vi "testIR.vi"() -> ()   [LabVIEW 2020]
uses:
  <vilib>/DAQmx/write.llb/DAQmx Write (Analog 2D DBL NChan NSamp).vi
  <vilib>/Utility/file.llb/Read Delimited Spreadsheet (DBL).vi
  <vilib>/DAQmx/miscellaneous.llb/DAQmx Fill In Error Info.vi
panel:
  out "Measured temperatures":dbl[](array[numeric])
  out "Input XY":i32[](array[numeric])
  in  "Desired temperature":dbl=30.0
  out "Input array":dbl[](array[numeric])
  in  "IR intensity value":dbl=10000.0
  in  "STIMULATE":bool
  out "Null Y output":dbl
  out "Null X output":dbl
  in  "LASER Intensity (%)":dbl=100.0 format="%#_13g"
  in  "Y input":i32=100
  in  "X input":i32=100
  out "Max. LASER Power (W)":dbl
  in  "Cycle Time (ms)":i32=50
  out "irData":dbl[](array[numeric])
  out "Temperature Measurements\n(Intensity Graph)":T1(graph)
  out "Intensity Graph":dbl[][](graph)
  out "Temperature array":dbl[][](array[numeric])
  in  "Temperature Range (High)":dbl=45.0
  in  "Temperature Range (Low)":dbl=20.0
  out "heatY":i32
  out "heatX":i32
  out "Deliver stimulation?":i32
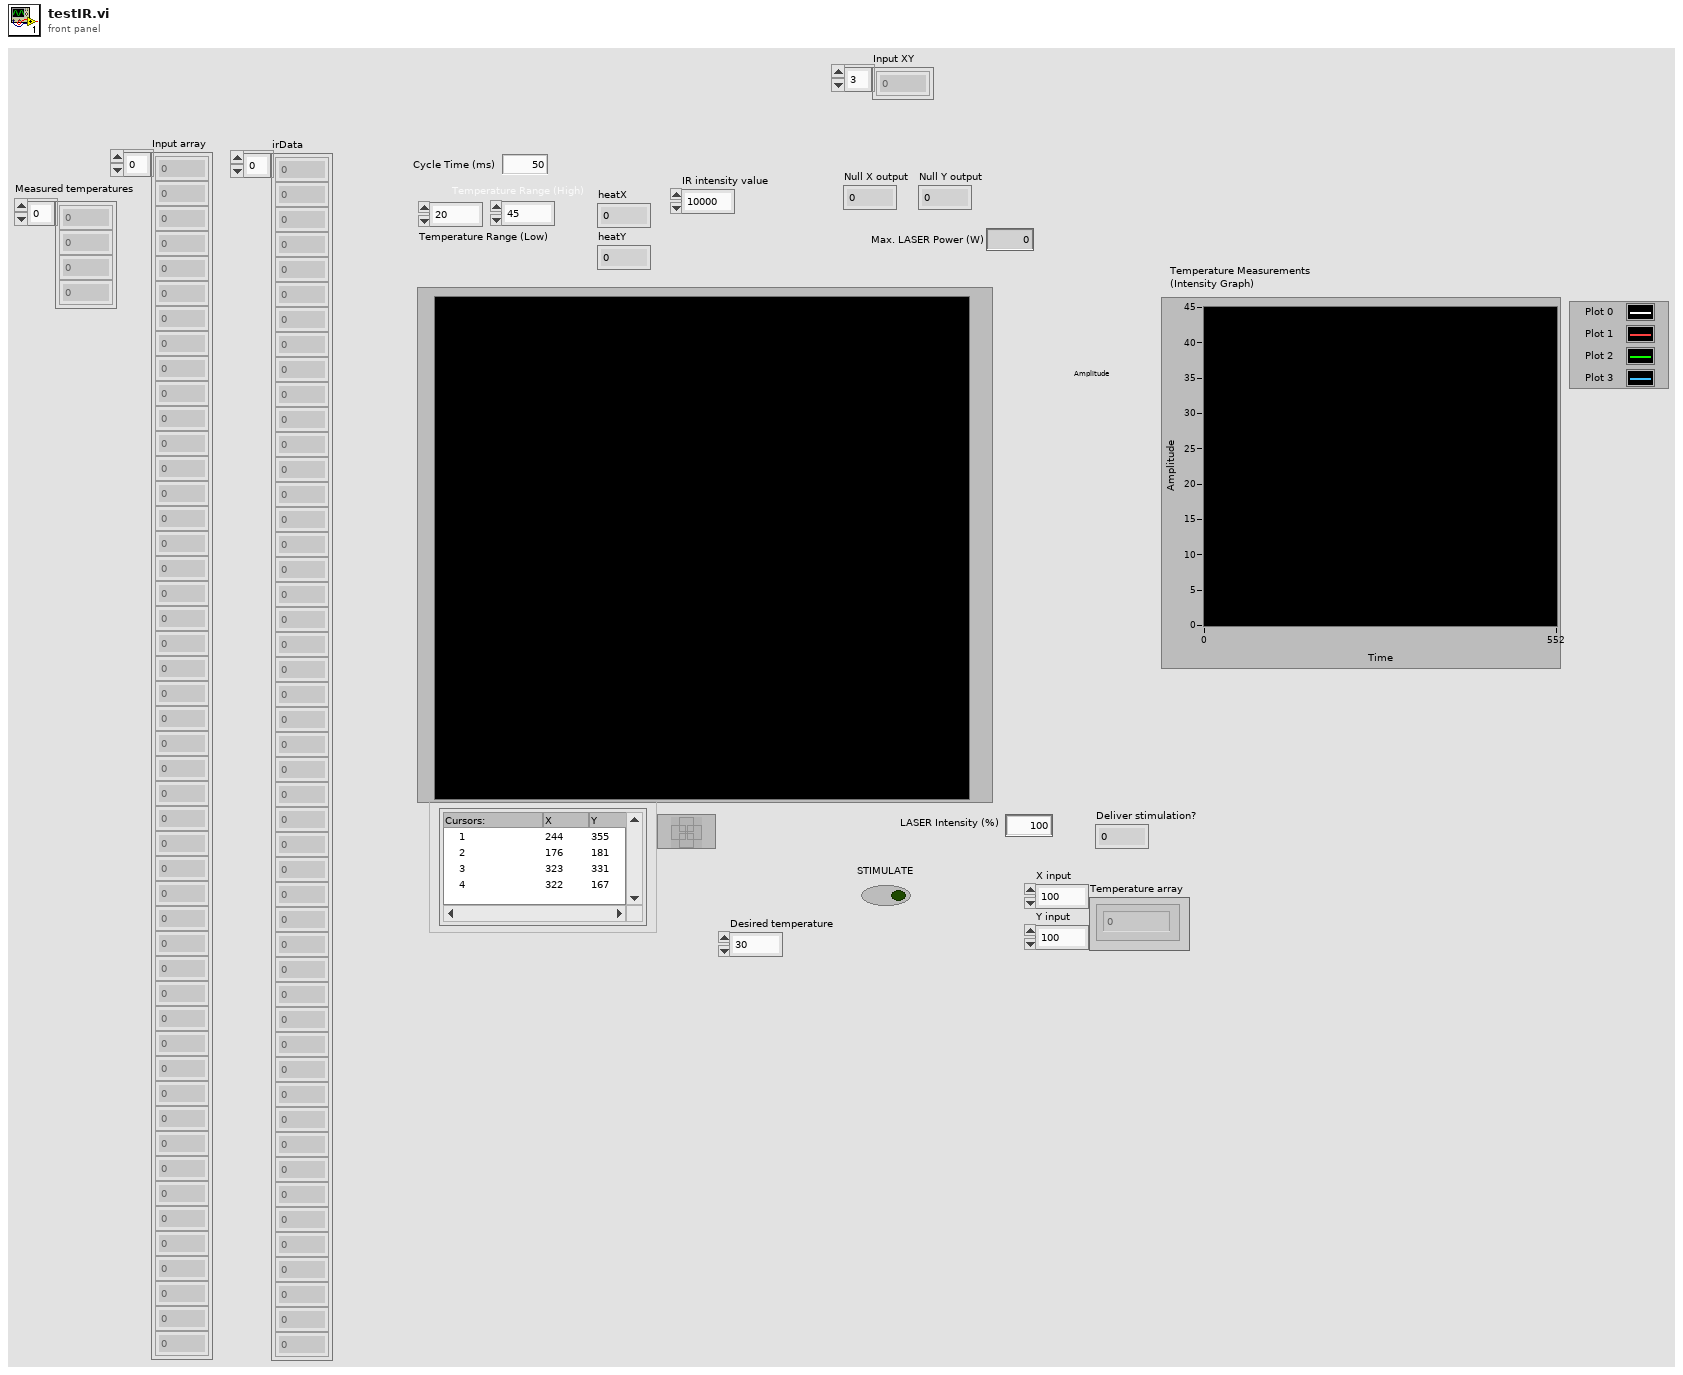
[diagram p1: front panel]
types:
  T1 = cluster{"[0]":dbl, "[1]":dbl, "[2]":dbl, "[3]":dbl, "[4]":dbl, "[5]":dbl, "[6]":dbl, "[7]":dbl, "[8]":dbl}
  T2 = enum16{"fire", "rainbow", "gray", "inverse gray", "ice", "original"}
  T3 = enum16{"open", "replace", "create", "open or create", "replace or create", "replace or create with confirmation"}
  T4 = enum16{"big-endian, network order", "native, host order", "little-endian"}
  T5 = typedef "IR GALVO Cal Data.ctl" = cluster{"G1X":dbl[][], "G1Y":dbl[][], "G2X":dbl[][], "G2Y":dbl[][], "G3X":dbl[][], "G3Y":dbl[][], "G4X":dbl[][], "G4Y":dbl[][], "G1 Intensity":dbl[][], "G2 Intensity":dbl[][], "G3 Intensity":dbl[][], "G4 Intensity":dbl[][], "L1 POWER":dbl[]}
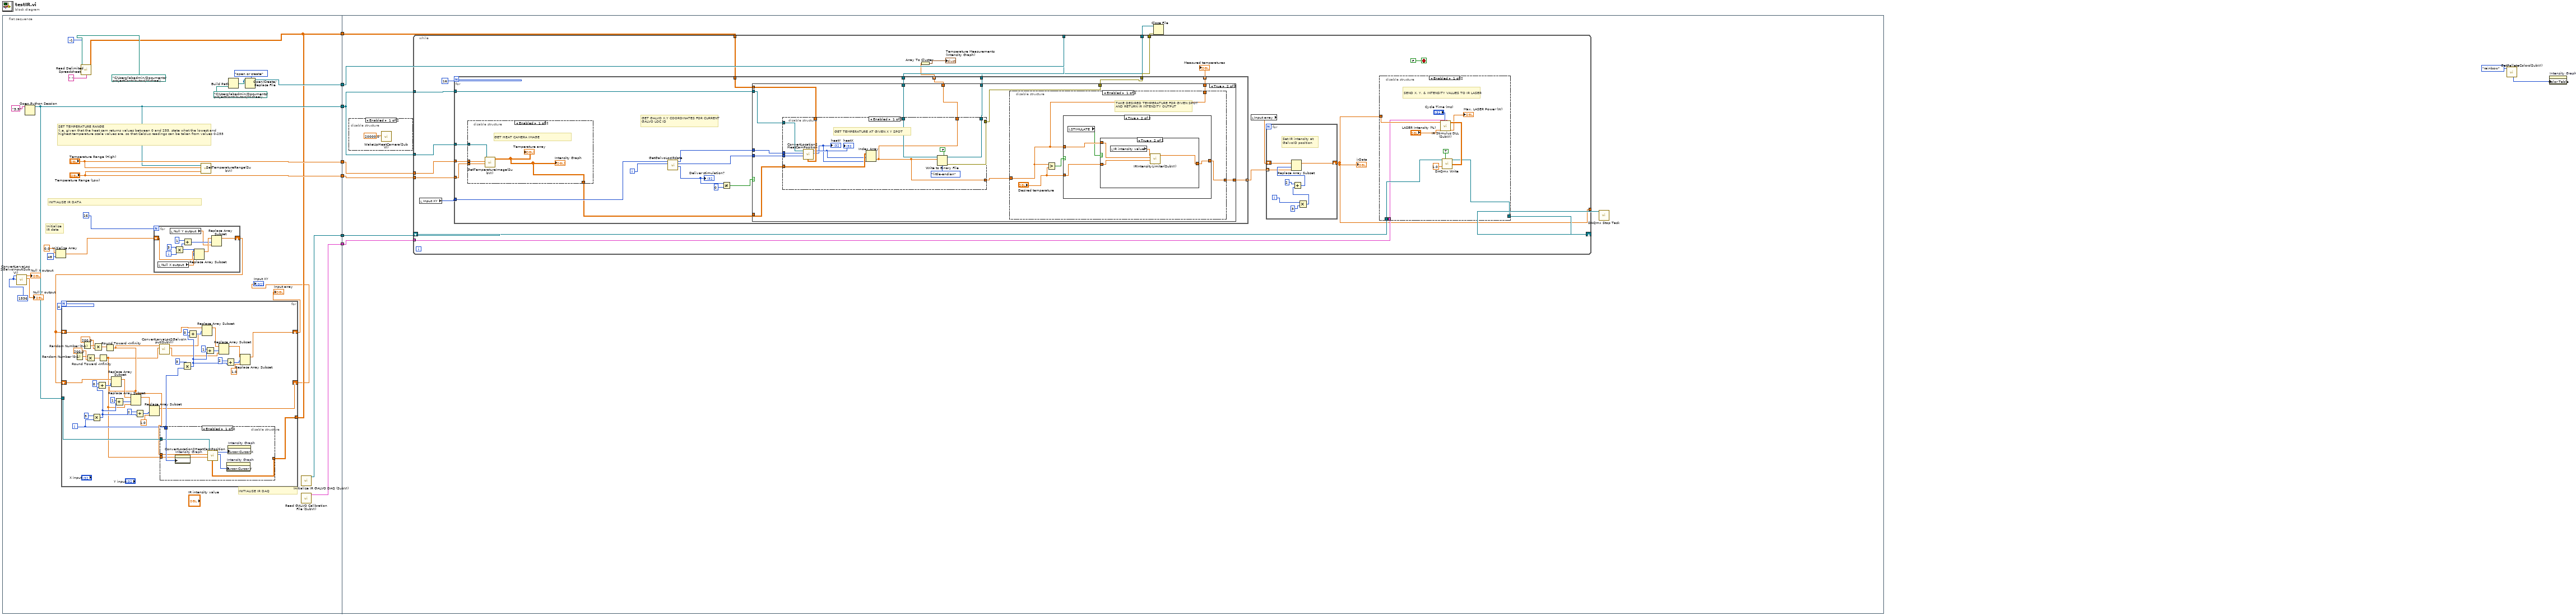
[diagram p0: block diagram]
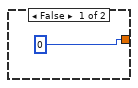
[diagram p4: hidden frame]
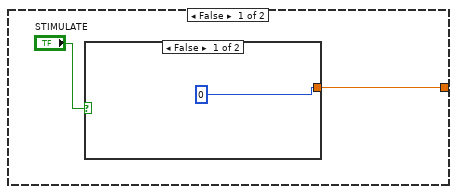
[diagram p6: hidden frame]
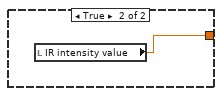
[diagram p7: hidden frame]
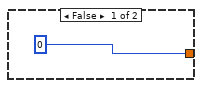
[diagram p8: hidden frame]
diagram:
  n1 = flat-sequence {
    tunnel: [w13] -> w7
    tunnel: ["Temperature Range (High)"] -> w6
    tunnel: ["Temperature Range (Low)"] -> w5
    tunnel: [w25] -> w4
    tunnel: [w23] -> w3
    tunnel: [w12] -> w2
    tunnel: [w16] -> w1
    tunnel: w7 -> [w93]
    tunnel: w6 -> [w92]
    tunnel: w5 -> [w91]
    tunnel: w4 -> [w99]
    tunnel: w3 -> [w98]
    tunnel: w2 -> [w97]
    tunnel: w1 -> [w96]
    frame #0 {
      w24 = 1536 ("X input")
      # "INITIALISE IR DAQ"
      # "INITIALISE IR DATA"
      # "SET TEMPERATURE RANGE\n(i.e. given that the heat cam returns values between 0 and 255, state what the lowest and highest temperature scale values are, so that Celsius readings can be taken from values 0-255"
      # "Initialise\nIR data"
      n2 = call "ConvertLarvaLoc2GalvoInput(SubVI).vi"("Y input"=w24, "X input"=w24) -> ("Y output"=→"Null Y output":dbl, "X output"=→"Null X output":dbl)  [unwired: 7 in, 1 out]
      n3 = Open Python Session(python version="3.9" ("Python version")) -> (session out=w13:refnum<k35>)  [unwired: 2 in, 1 out]
      n4 = Initialize Array(0.0 ("element"), 48 ("dimension size")) -> (w33:dbl[])
      n5 = call-poly <vilib>:"Read Delimited Spreadsheet.vi"("file path (dialog if empty)"=path "C:/Users/labadmin/Documents/projectContributors/Michael/multi-larva-cl-behavior-detection/LabViewSourceCode/heatCameraPythonCode/transformationMatrix.csv", "number of rows (all:-1)"=-1, "delimiter (\\t)"=" " ("delimiter (\\t)")) -> ("all rows"=w12:dbl[][])  [unwired: 7 in, 5 out]
      n6 = for {
        N: 16 -> [_]
        shift-right: [w37] -> w11
        shift-left: w33 -> [w41]
        i -> [w43]
        n7 = local read "Null X output"() -> (w36:dbl)
        n8 = local read "Null Y output"() -> (w35:dbl)
        n9 = Multiply(x=3, y=w43) -> (x*y=w40:i32)
        n10 = Add(x=1, y=w40) -> (x+y=w38:i32)
        n11 = Replace Array Subset(array=w41, new element=w36, index=w40) -> (w39:dbl[])
        n12 = Replace Array Subset(array=w39, new element=w35, index=w38) -> (w37:dbl[])
      }
      n13 = for {
        N: 4 -> [_]
        shift-right: [w82] -> w15
        shift-left: w11 -> [w79]
        tunnel: w13 -> [w66]
        tunnel: w12 -> [w61]
        shift-right: [w46] -> w10
        shift-left: w11 -> [w50]
        i -> [w48]
        n14 = Random Number (0-1)() -> (number: 0 to 1=w67:dbl)
        n15 = Random Number (0-1)() -> (number: 0 to 1=w70:dbl)
        n16 = Multiply(x=w67, y=200.0) -> (x*y=w65:dbl)
        n17 = Multiply(x=3, y=w48) -> (x*y=w59:i32)
        n18 = Multiply(x=w70, y=200.0) -> (x*y=w64:dbl)
        n19 = Add(x=0, y=w59) -> (x+y=w54:i32)
        n20 = Round Toward -Infinity(1:w65) -> (0:w45:dbl)
        n21 = Round Toward -Infinity(1:w64) -> (0:w49:dbl)
        n22 = Replace Array Subset(array=w50, new element=w49, index=w54) -> (w51:dbl[])
        n23 = Add(x=1, y=w59) -> (x+y=w56:i32)
        n24 = Replace Array Subset(array=w51, new element=w45, index=w56) -> (w52:dbl[])
        n25 = Add(x=2, y=w59) -> (x+y=w58:i32)
        n26 = Replace Array Subset(array=w52, new element=1.0 ("new element/subarray"), index=w58) -> (w46:dbl[])
        n27 = call "ConvertLarvaLoc2GalvoInput(SubVI).vi"("Y input"=w45, "X input"=w49) -> ("Y output"=w62:dbl, "X output"=w63:dbl)  [unwired: 7 in, 1 out]
        n28 = disable-structure shown="Enabled" {
          disable-tunnel: w48 -> [w90 _]
          disable-tunnel: w66 -> [w89 _]
          disable-tunnel: w61 -> [w86 _]
          disable-tunnel: w49 -> [w85 _]
          disable-tunnel: w45 -> [w84 _]
          frame Enabled {
            n29 = property on="Intensity Graph" class="IntGraph (strict)"("Active Cursor"=w90) -> ()  [unwired: 2 in, 2 out]
            n30 = call "ConvertLocation2HeatCamPosition.vi"("Transformation matrix"=w86, "yLoc"=w84, "xLoc"=w85, "Python session"=w89) -> ("Heat cam Y"=w87:i32, "Heat cam X"=w88:i32)  [unwired: 6 in]
            n31 = property on="Intensity Graph" class="IntGraph (strict)"("Cursor.Cursor Y"=w87) -> ()  [unwired: 2 in, 2 out]
            n32 = property on="Intensity Graph" class="IntGraph (strict)"("Cursor.Cursor X"=w88) -> ()  [unwired: 2 in, 2 out]
          }
          frame Disabled {
          }
        }
        n33 = Multiply(x=3, y=w48) -> (x*y=w72:i32)
        n34 = Add(x=0, y=w72) -> (x+y=w77:i32)
        n35 = Replace Array Subset(array=w79, new element=w63, index=w77) -> (w83:dbl[])
        n36 = Add(x=1, y=w72) -> (x+y=w75:i32)
        n37 = Replace Array Subset(array=w83, new element=w62, index=w75) -> (w81:dbl[])
        n38 = Add(x=2, y=w72) -> (x+y=w73:i32)
        n39 = Replace Array Subset(array=w81, new element=1.0 ("new element/subarray"), index=w73) -> (w82:dbl[])
      }
      "Input array" <- w15
      "Input XY" <- w10
      n40 = call "SetTemperatureRange(SubVI).vi"("Temperature Range (Low) in"="Temperature Range (Low)", "Temperature Range (High) in"="Temperature Range (High)", "Refnum in"=w13) -> ()  [unwired: 9 in]
      n41 = Build Path(name or relative path=path "C:/Users/labadmin/Documents/projectContributors/Michael/multi-larva-cl-behavior-detection/LabViewSourceCode/heatCameraPythonCode/outputData.bin" ("file path (dialog if empty)")) -> (appended path=w19:path)  [unwired: 1 in]
      n42 = Open/Create/Replace File(file path (use dialog)=w19, operation (0:open)=T3."open or create") -> (refnum out=w16:refnum<file>)  [unwired: 4 in, 2 out]
      n43 = call "Initialize IR GALVO DAQ (SubVI).vi"() -> ("Refnum out"=w25:refnum<k21>)  [unwired: 11 in]
      n44 = call "Read GALVO Calibration File (SubVI).vi"() -> ("GALVO Cal Data"=w23:T5)  [unwired: 11 in]
    }
    frame #1 {
      n45 = disable-structure shown="Enabled" {
        frame Enabled {
          n46 = call "WakeUpHeatCamera(SubVI).vi"("Time (ms) to wait"=20000.0) -> ()  [unwired: 11 in]
        }
        frame Disabled {
        }
      }
      n47 = while {
        tunnel: w93 -> [w120]
        tunnel: w98 -> [w109]
        tunnel: w97 -> [w119]
        tunnel: w96 -> [w118]
        shift-right: [w108] -> w100
        shift-left: w99 -> [w110]
        tunnel: [w116] -> w95
        tunnel: [w115] -> w94
        tunnel: w93 -> [w113]
        tunnel: w92 -> [w112]
        tunnel: w91 -> [w111]
        tunnel: [w106] -> _
        stop <- FALSE stop-if-true
        n48 = local read "Input XY"() -> (w104:i32[])
        n49 = for {
          N: 16 -> [_]
          tunnel: w120 -> [w157]
          tunnel: [w156] -> w116
          tunnel: w119 -> [w155]
          tunnel: w118 -> [w154]
          tunnel: [w152] -> w115
          tunnel: w113 -> [w151]
          tunnel: w112 -> [w150]
          tunnel: w111 -> [w149]
          tunnel: w104 -> [w153]
          tunnel: [w145] -> w107 mode=indexing
          tunnel: [w140] -> w103 mode=indexing
          tunnel: [w139] -> w101 mode=indexing
          i -> [w144]
          # "GET GALVO X,Y COORDINATES FOR CURRENT GALVO LOC ID"
          n50 = disable-structure shown="Enabled" {
            disable-tunnel: w151 -> [w204 _]
            disable-tunnel: w150 -> [w203 _]
            disable-tunnel: w149 -> [w202 _]
            disable-tunnel: [w201 _] -> w148
            frame Enabled {
              # "GET HEAT CAMERA IMAGE"
              n51 = call "GetTemperatureImage(SubVI).vi"("Refnum in"=w204, "Temperature Range (High)"=w203, "Temperature Range (Low)"=w202) -> ("Temperature array out"=w201:dbl[][])  [unwired: 7 in]
              "Temperature array" <- w201
              "Intensity Graph" <- w201
            }
            frame Disabled {
            }
          }
          n52 = call "GetGalvoLocIRdata.vi"("Galvo location"=w144, "irData"=w153) -> ("temperature"=w141:i32, "yLoc"=w146:i32, "xLoc"=w147:i32)  [unwired: 7 in]
          "Deliver stimulation?" <- w141
          n53 = Not Equal?(x=w141, y=0) -> (x != y?=w142:bool)
          n54 = case shown="True" w142 {
            tunnel: w157 -> [_ w170]
            tunnel: [_ w168] -> w156
            tunnel: w155 -> [_ w167]
            tunnel: w154 -> [_ w166]
            tunnel: [_ w165] -> w152
            tunnel: w148 -> [_ w164]
            tunnel: w147 -> [_ w163]
            tunnel: w146 -> [_ w162]
            tunnel: [0 w161] -> w145
            tunnel: [_ w160] -> w140
            tunnel: [_ w159] -> w139
            frame False {
            }
            frame True {
              n55 = disable-structure shown="Enabled" {
                disable-tunnel: w163 -> [w183 _]
                disable-tunnel: w162 -> [w182 _]
                disable-tunnel: w170 -> [w181 _]
                disable-tunnel: w164 -> [w180 _]
                disable-tunnel: [w173 _] -> w169
                disable-tunnel: [w179 _] -> w168
                disable-tunnel: w167 -> [w178 _]
                disable-tunnel: w166 -> [w177 _]
                disable-tunnel: [w174 _] -> w165
                disable-tunnel: [w173 _] -> w160
                frame Enabled {
                  # "GET TEMPERATURE AT GIVEN X Y SPOT"
                  n56 = call "ConvertLocation2HeatCamPosition.vi"("Transformation matrix"=w178, "yLoc"=w182, "xLoc"=w183, "Python session"=w181) -> ("Heat cam Y"=w171:i32, "Heat cam X"=w172:i32)  [unwired: 6 in]
                  "heatX" <- w172
                  "heatY" <- w171
                  n57 = Index Array(array=w180, index (row)=w172, index (col)=w171) -> (element=w173:dbl)
                  n58 = Write to Binary File(file (use dialog)=w177, data=w173, 5:FALSE ("prepend array or string size? (T)"), 9:T4."little-endian" ("byte order (0:big-endian, network order)")) -> (refnum out=w174:refnum<file>, error out=w179:errorcluster)  [unwired: 2 in, 1 out]
                }
                frame Disabled {
                }
              }
              n59 = disable-structure shown="Enabled" {
                disable-tunnel: w169 -> [w184 _]
                disable-tunnel: [w186 _] -> w161
                disable-tunnel: [w184 _] -> w159
                frame Enabled {
                  # "TAKE DESIRED TEMPERATURE FOR GIVEN SPOT AND RETURN IR INTENSITY OUTPUT"
                  n60 = Greater?(x=w184, y="Desired temperature") -> (0:w187:bool)
                  n61 = case shown="True" w187 {
                    tunnel: [w188 w193] -> w186
                    tunnel: "Desired temperature" -> [_ w194]
                    tunnel: w184 -> [_ w195]
                    frame False {
                      n62 = case shown="False" "STIMULATE" {
                        tunnel: [0 ("index") w191] -> w188
                        frame False {
                        }
                        frame True {
                          n63 = local read "IR intensity value"() -> (w191:dbl)
                        }
                      }
                    }
                    frame True {
                      n64 = local read "STIMULATE"() -> (w192:bool)
                      n65 = case shown="True" w192 {
                        tunnel: w195 -> [_ w200]
                        tunnel: w194 -> [_ w198]
                        tunnel: [0 ("index") w197] -> w193
                        frame False {
                        }
                        frame True {
                          n66 = local read "IR intensity value"() -> (w199:dbl)
                          n67 = call "IRIntensityLimiter(SubVI).vi"("Desired temperature"=w198, "Current temperature"=w200, "Maximum intensity"=w199) -> ("Intensity output"=w197:dbl)  [unwired: 8 in]
                        }
                      }
                    }
                  }
                }
                frame Disabled {
                }
              }
            }
          }
        }
        "Measured temperatures" <- w101
        n68 = Array To Cluster(array=w103) -> (cluster=→"Temperature Measurements\n(Intensity Graph)":T1)
        n69 = local read "Input array"() -> (w105:dbl[])
        n70 = for {
          tunnel: w107 -> [w124] mode=indexing
          shift-right: [w122] -> w106
          shift-left: w105 -> [w123]
          i -> [w121]
          # "Set IR intensity at GalvoID position"
          n71 = Multiply(x=w121, y=3 ("index")) -> (x*y=w127:i32)
          n72 = Add(x=2 ("index"), y=w127) -> (x+y=w128:i32)
          n73 = Replace Array Subset(array=w123, new element=w124, index=w128) -> (w122:dbl[])
        }
        "irData" <- w106
        n74 = disable-structure shown="Enabled" {
          disable-tunnel: w110 -> [w137 _]
          disable-tunnel: [w136 _] -> w108
          disable-tunnel: w106 -> [w131 _]
          disable-tunnel: w109 -> [w129 _]
          frame Enabled {
            # "SEND X, Y, & INTENSITY VALUES TO IR LASER"
            n75 = call "IR Stimulus DLL (SubVI).vi"("GALVO Calibration Data"=w129, "Cycle Time (ms)"="Cycle Time (ms)", "LASER Intensity (%)"="LASER Intensity (%)", "irData"=w131) -> ("Max. LASER Power (W)"=→"Max. LASER Power (W)":dbl, "daqData"=w138:dbl[][])  [unwired: 6 in]
            n76 = call-poly <vilib>:"DAQmx Write.vi"("task/channels in"=w137, "auto start"=TRUE, "data"=w138, "timeout"=1.0) -> ("task out"=w136:refnum<k21>)  [unwired: 9 in, 2 out]
          }
          frame Disabled {
          }
        }
      }
      n77 = Close File(refnum=w94, error in=w95) -> ()  [unwired: 2 out]
      n78 = call <vilib>:"DAQmx Stop Task.vi"("task/channels in"=w100) -> ()  [unwired: 13 in, 2 out]
    }
  }
  n79 = call "GetPalleteColors(SubVI).vi"("Map Selector"=T2."rainbow") -> ("Map output"=w8:u32[])  [unwired: 10 in]
  n80 = property on="Intensity Graph" class="IntGraph (strict)"("Color Table"=w8) -> ()  [unwired: 2 in, 2 out]
